vi "Delete Item.vi"(8 "error in (no error)":errorcluster, 10 "Removed VI":refnum<class "Standard VI Type.lvclass">, 11 "Data in":T1) -> (0 "error out":errorcluster, 3 "Data out":T1)   [LabVIEW 2020, in "Peek Window.lvlib"]
uses:
  Peek Window.lvlib
  MHL Data Cluster.ctl
  VI Types/Standard VI Type/Standard VI Type.lvclass
  VI Types/Standard VI Type/Standard VI Type.lvclass/Standard VI Type.ctl
  VI Types/Standard VI Type/Read Full Qualified Name.vi
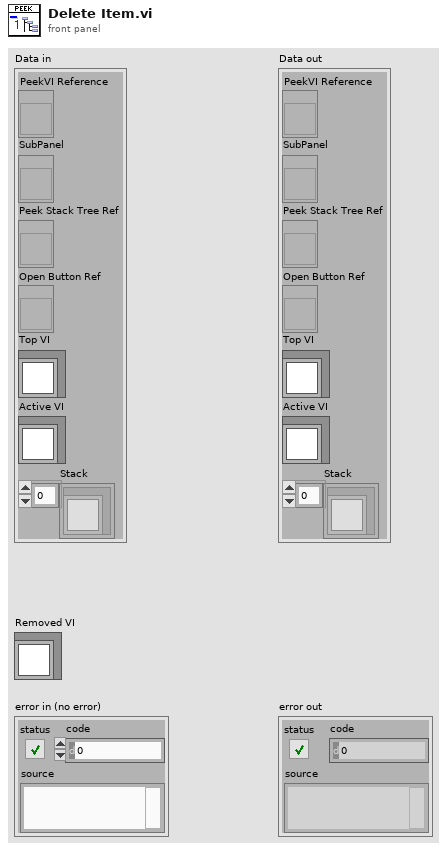
[diagram p1: front panel]
types:
  T1 = typedef "Peek Window.lvlib/MHL Data Cluster.ctl" = cluster{"PeekVI Reference":refnum<vi>, "SubPanel":refnum<vi>, "Peek Stack Tree Ref":refnum<vi>, "Open Button Ref":refnum<vi>, "Top VI":refnum<class "Standard VI Type.lvclass">, "Active VI":refnum<class "Standard VI Type.lvclass">, "Stack":refnum<class "Standard VI Type.lvclass">[]}
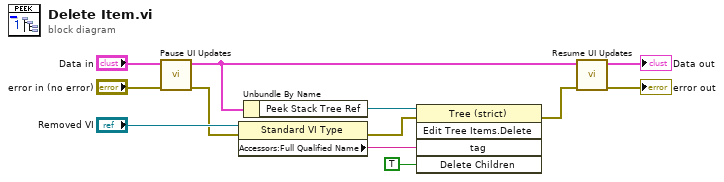
[diagram p0: block diagram]
diagram:
  n1 = call "Pause UI Updates.vi"("error in"="error in (no error)", "Module Data"="Data in") -> ("error out"=w2:errorcluster, "Module Data"=w6:T1)  [unwired: 8 in]
  n2 = property class="Standard VI Type"(reference="Removed VI", error in=w2) -> (error out=w1:errorcluster, "Accessors:Full Qualified Name"=w3:string)  [unwired: 1 out]
  n3 = Unbundle By Name(w6) -> ("Peek Stack Tree Ref"=w12:refnum<vi>)
  n4 = invoke class="Tree (strict)" method="Edit Tree Items.Delete"(reference=w12, error in=w1, "tag"=w3, "Delete Children"=TRUE) -> (error out=w5:errorcluster)  [unwired: 1 in, 4 out]
  n5 = call "Resume UI Updates.vi"("error in"=w5, "Module Data"=w6) -> ("error out"=→"error out":errorcluster, "Module Data"=→"Data out":T1)  [unwired: 8 in]
